vi "Memory.Truncate I64.vi"(11 "I64":i64) -> (3 "truncated I64":i64)   [LabVIEW 2016, in "LabVIEW Memory Manager.lvlib"]
uses:
  LabVIEW Memory Manager.lvlib
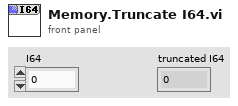
[diagram p1: front panel]
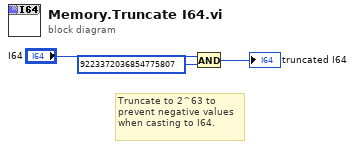
[diagram p0: block diagram]
diagram:
  # "Truncate to 2^63 to prevent negative values when casting to I64."
  n1 = And(x="I64", y=i64 9223372036854775807) -> (x .and. y?=→"truncated I64":i64)
